vi "CCMWLQuery.vi"(8 "error in (no error)":errorcluster) -> (0 "error out":errorcluster, 1 "Cancel?":bool, 2 "Worklist":string[][](table), 3 "subarray":string[](array[string]))   [LabVIEW 2013, in "main.lvlib" / "ClearCanvasLibrary.lvlib"]
uses:
  ClearCanvasLibrary.lvlib
  <userlib>/_MGI/Error Handling/MGI Suppress Error Code/MGI Suppress Error Code (Scalar).vi
  <vilib>/Utility/cursorutil.llb/Set Cursor (Icon Pict).vi
  <vilib>/Utility/miscctls.llb/LVRowAndColumnTypeDef.ctl
  main.lvlib
  Controls/Enum Save Action Events.ctl
  Controls/SaveDataCluster.ctl
panel:
  in  "TimeEnd":timestamp caption="End" format="%<%x>T"
  in  "TimeStart":timestamp caption="Start" format="%<%x>T"
  in  "SelectPatient":bool
  out "VerificationSCU":bool
  in  "Exit":bool
  in  "queryWorklist":bool
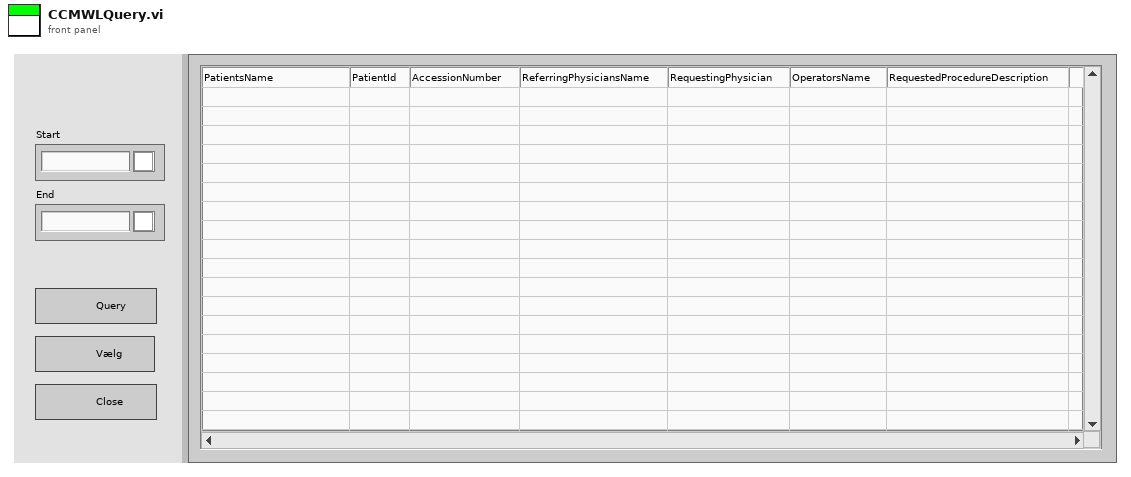
[diagram p1: front panel]
types:
  T1 = typedef "main.lvlib/SaveDataCluster.ctl" = cluster{"HospInfo":cluster{"Name":string, "Address":string, "Department":string}, "Pressure":cluster{"Pressure":dbl}, "DataPath":cluster{"DataPath":path}, "ReportPath":cluster{"Path":path, "Name":string}, "DICOM Info WL":cluster{"port":i32, "AEtitle":string, "host":string, "remoteAE":string}, "DICOM Info PACS":cluster{"port":i32, "AEtitle":string, "host":string, "remoteAE":string}, "ArmCalcMethod":dbl, "itemTags":string[], "DicomEncoding":u16, "JournalType":u16, "General Settings":cluster{"Hyphenation":bool, "Language":u16, "CellStr1":string, "CellStr2":string}, "Dicom Tags":string[][], "BT Serial":cluster{"Serial Number":string, "Side":string, "Ignore?":bool}[], "BT License":cluster{"License":string, "Accepted Serials":string[]}}
  T2 = typedef "main.lvlib/Enum Save Action Events.ctl" = enum16{"LoadReportPath", "SaveReportPath", "Load Graph Path", "Save Graph Path", "LoadDataPath", "SaveDataPath", "Load Template Path", "Save Template Path", "Load PressureFactor", "Save PressureFactor", "Init", "Load Listbox", "Save Listbox", "LoadHospInfo", "SaveHospInfo", "Load DICOM Activation", "Save DICOM Activation", "LoadDICOMInfoWL", "SaveDICOMInfoWL", "LoadDICOMInfoPACS", "SaveDICOMInfoPACS", "Load ArmCalcMethod", "Save ArmCalcMethod", "LoadItemTags", "SaveItemTags", "LoadDICOMEncoding", "SaveDICOMEncoding", "LoadJournalType", "SaveJournalType", "LoadAcqFilterType", "SaveAcqFilterType", "Load Sequence", "Save Sequence", "Load Acquisition Mode", "Save Acquisition Mode", "Load General Settings", "Save General Settings", "Load Language", "Save Language", "Load Dicom Tags", "Save Dicom Tags", "Load BT Serial", "Save BT Serial", "Load BT License", "Save BT License"}
  T3 = typedef "LVRowAndColumnTypeDef.ctl" = cluster{"Row":i32, "Column":i32}
  T4 = cluster{"port":i32, "AEtitle":string, "host":string, "remoteAE":string}
  T5 = cluster{"TimeStart":timestamp, "TimeEnd":timestamp}
  T6 = typedef "LVPoint32TypeDef.ctl" = cluster{"Horizontal":i32, "Vertical":i32}
  T7 = cluster{"port":i32, "AEtitle":string, "remoteAE":string, "host":string}
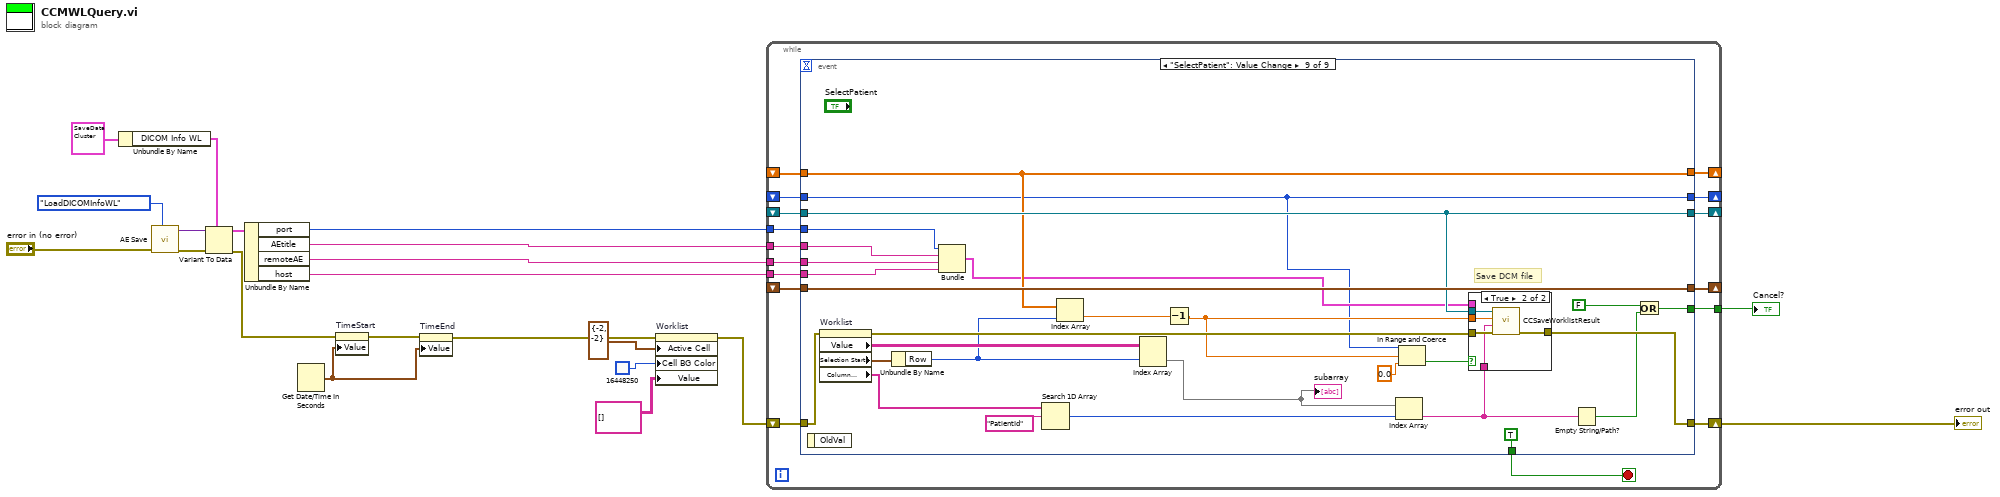
[diagram p0: block diagram]
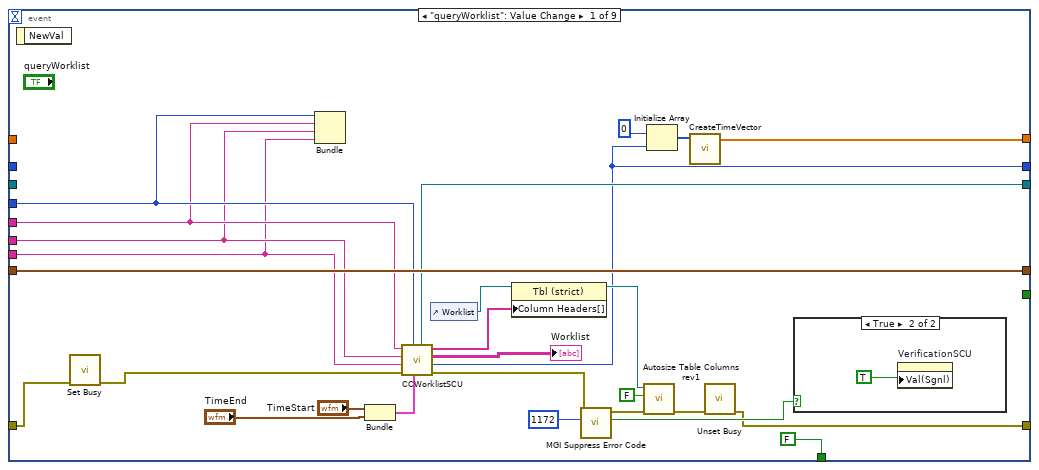
[diagram p2: hidden frame]
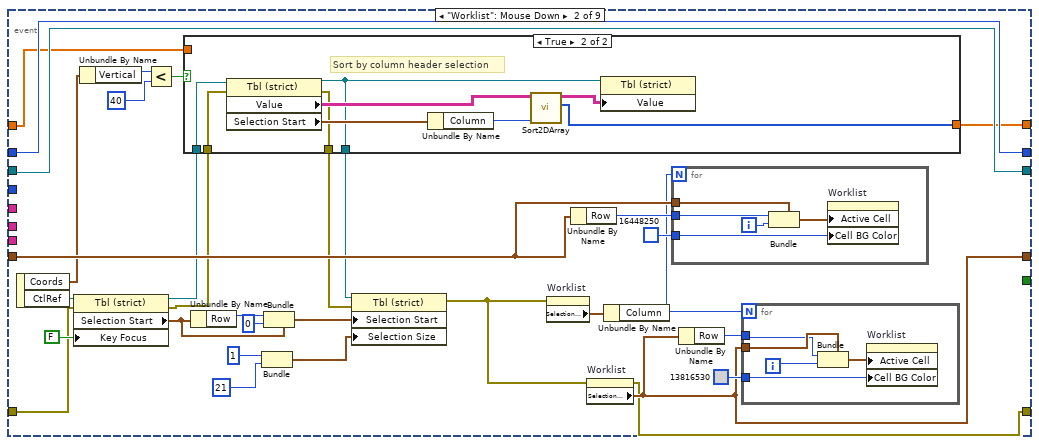
[diagram p4: hidden frame]
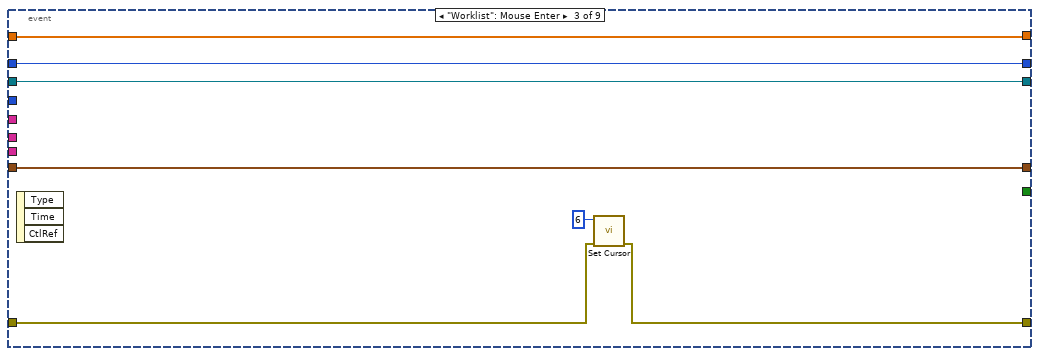
[diagram p6: hidden frame]
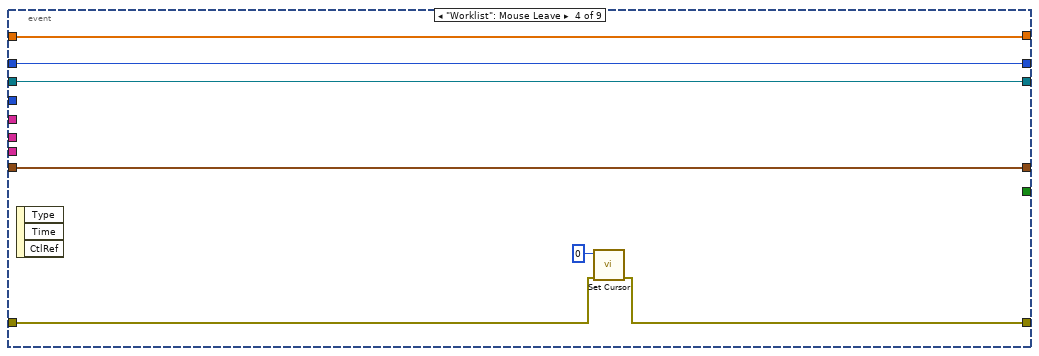
[diagram p7: hidden frame]
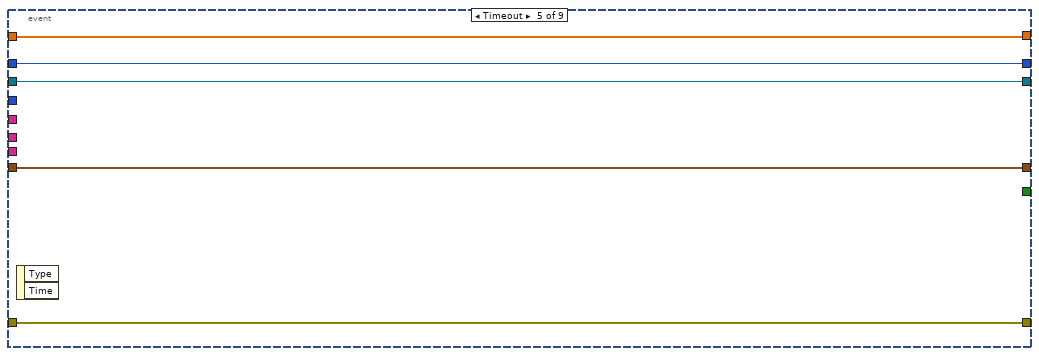
[diagram p8: hidden frame]
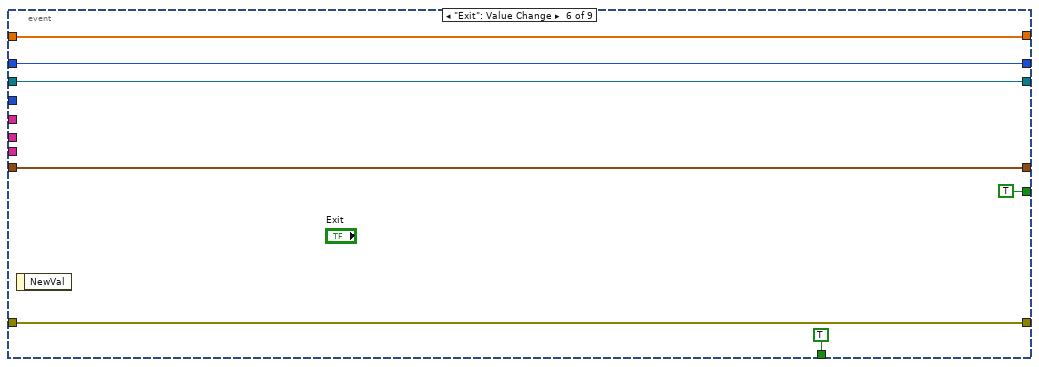
[diagram p9: hidden frame]
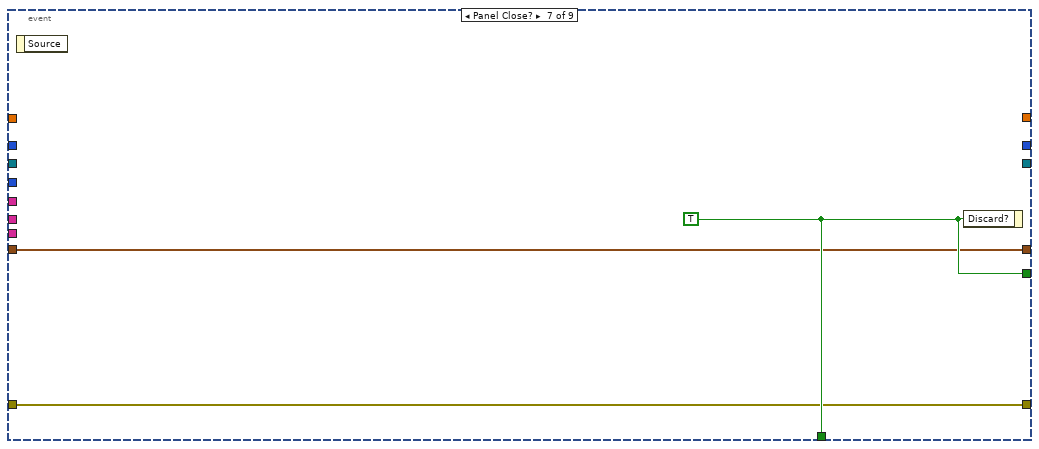
[diagram p10: hidden frame]
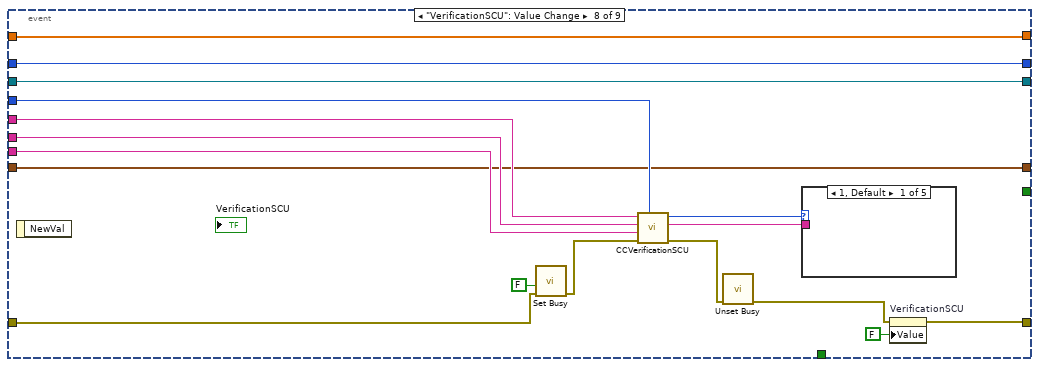
[diagram p11: hidden frame]
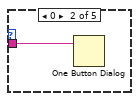
[diagram p12: hidden frame]
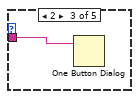
[diagram p13: hidden frame]
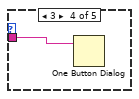
[diagram p14: hidden frame]
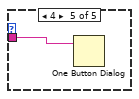
[diagram p15: hidden frame]
diagram:
  n1 = Unbundle By Name(T1 {"HospInfo"={"Name"="", "Address"="", "Department"=""}, "Pressure"={"Pressure"=0.0}, "DataPath"={"DataPath"=path ""}, "ReportPath"={"Path"=path "", "Name"=""}, "DICOM Info WL"={"port"=0, "AEtitle"="", "host"="", "remoteAE"=""}, "DICOM Info PACS"={"port"=0, "AEtitle"="", "host"="", "remoteAE"=""}, "ArmCalcMethod"=0.0, "itemTags"=[], "DicomEncoding"=0, "JournalType"=0, "General Settings"={"Hyphenation"=FALSE, "Language"=0, "CellStr1"="", "CellStr2"=""}, "Dicom Tags"=[], "BT Serial"=[], "BT License"={"License"="", "Accepted Serials"=[]}} ("Data")) -> ("DICOM Info WL"=w11:T4)
  n2 = call "AE Save.vi"("error in (no error)"="error in (no error)", "Action"=Enum_Save_Action_Events."LoadDICOMInfoWL") -> ("error out"=w12:errorcluster, "Anything"=w16:variant)  [unwired: 7 in]
  n3 = Variant To Data(error in=w12, type=w11, Variant=w16) -> (data=w14:T4, error out=w5:errorcluster)
  n4 = Unbundle By Name(w14) -> ("port"=w9:i32, "AEtitle"=w8:string, "remoteAE"=w7:string, "host"=w6:string)
  n5 = Get Date/Time In Seconds() -> (seconds since 1Jan1904=w2:timestamp)
  n6 = property on="TimeStart" class="AbsTime (strict)"(error in=w5, "Value"=w2) -> (error out=w4:errorcluster)  [unwired: 1 in, 1 out]
  n7 = property on="TimeEnd" class="AbsTime (strict)"(error in=w4, "Value"=w2) -> (error out=w3:errorcluster)  [unwired: 1 in, 1 out]
  n8 = property on="Worklist" class="Tbl (strict)"(error in=w3, "Active Cell"=T3 {"Row"=-2, "Column"=-2} ("Active Cell:Active Cell"), "Cell BG Color"=u32 16448250, "Value"=string[][] [] ("Worklist")) -> (error out=w19:errorcluster)  [unwired: 1 in, 1 out]
  n9 = while {
    shift-right: [w36] -> _
    shift-left: _ -> [w35]
    shift-right: [w33] -> w10
    shift-left: w19 -> [w34]
    shift-right: [w32] -> _
    shift-left: _ -> [w31]
    shift-right: [w30] -> _
    shift-left: _ -> [w29]
    tunnel: w9 -> [w28]
    tunnel: w8 -> [w27]
    tunnel: w7 -> [w26]
    tunnel: w6 -> [w25]
    shift-right: [w24] -> _
    shift-left: _ -> [w23]
    tunnel: [w22] -> w1
    stop <- w37 stop-if-true
    n10 = event shown="[8] \"SelectPatient\": Value Change" {
      selector: _ -> [_ _ _ _ _ _ _ _ _]
      dyn-events: _ -> [_ _ _ _ _ _ _ _ _]
      timeout: _ -> [_ _ _ _ _ _ _ _ _]
      tunnel: [FALSE _ _ _ _ TRUE w148 _ TRUE] -> w37
      tunnel: w25 -> [w38 _ _ _ _ _ _ w157 w173]
      tunnel: w26 -> [w39 _ _ _ _ _ _ w158 w172]
      tunnel: w27 -> [w40 _ _ _ _ _ _ w159 w174]
      tunnel: w28 -> [w41 _ _ _ _ _ _ w160 w175]
      tunnel: [w59 w93 w125 w132 w138 w144 w146 w154 w196] -> w36
      tunnel: w35 -> [w59 w92 w125 w132 w138 w144 w146 w154 w196]
      tunnel: w34 -> [w58 w81 w124 w131 w137 w143 w147 w153 w194]
      tunnel: [w57 w80 w123 w130 w137 w143 w147 w152 w191] -> w33
      tunnel: [w56 w79 w122 w129 w136 w142 _ w151 w193] -> w32
      tunnel: w31 -> [_ w79 w122 w129 w136 w142 _ w151 w193]
      tunnel: [w44 w78 w121 w128 w135 w141 _ w150 w170] -> w30
      tunnel: w29 -> [_ w78 w121 w128 w135 w141 _ w150 w170]
      tunnel: [w42 w69 w120 w127 w134 w140 _ w149 w183] -> w24
      tunnel: w23 -> [_ w68 w120 w127 w134 w140 _ w149 w183]
      tunnel: [_ _ _ _ _ TRUE w148 _ w178] -> w22
      event "queryWorklist": Value Change {
        n11 = event-data() -> ()  [unwired: 1 in, 1 out]
        n12 = call <vilib>:"Set Busy.vi"("error in (no error)"=w58) -> ("error out"=w61:errorcluster)  [unwired: 9 in, 1 out]
        n13 = Bundle("port"=w41, "AEtitle"=w40, "remoteAE"=w39, "host"=w38) -> ()  [unwired: 1 in, 1 out]
        n14 = Bundle("TimeStart"="TimeStart", "TimeEnd"="TimeEnd") -> (w55:T5)  [unwired: 1 in]
        n15 = call "CCWorklistSCU.vi"("TimeCluster"=w55, "remotePort"=w41, "error in (no error)"=w61, "remoteHost"=w38, "remoteAE"=w39, "clientAETitle"=w40) -> ("error out"=w60:errorcluster, "patientsRetrieved"=w44:i32, "Worklist"=→"Worklist":string[][], "DicomTags"=w47:string[], "Find"=w56:refnum<k24>)  [unwired: 1 in]
        n16 = control-ref of="Worklist"() -> (w48:refnum<vi>)
        n17 = property class="Tbl (strict)"(reference=w48, "Column Headers[]"=w47) -> (reference out=w46:refnum<vi>)  [unwired: 1 in, 1 out]
        n18 = call-poly <userlib>:"MGI Suppress Error Code.vi"("Error Code"=1172, "Error In"=w60) -> ("Error Supressed?"=w62:bool, "Error Out"=w50:errorcluster)  [unwired: 4 in]
        n19 = call "Autosize Table Columns rev1.vi"("error in (no error)"=w50, "Resize Table?"=FALSE, "Table Ref"=w46) -> ("error out"=w51:errorcluster)  [unwired: 4 in]
        n20 = Initialize Array(0 ("dimension size"), w44) -> (w43:i32[])
        n21 = call "CreateTimeVector.vi"("Array in"=w43) -> ("Array out"=w42:dbl[])  [unwired: 10 in]
        n22 = call <vilib>:"Unset Busy.vi"("error in (no error)"=w51) -> ("error out"=w57:errorcluster)  [unwired: 10 in]
        n23 = case shown="True" w62 {
          frame False {
          }
          frame True {
            n24 = property on="VerificationSCU" class="Bool (strict)"("Val(Sgnl)"=TRUE) -> ()  [unwired: 2 in, 2 out]
          }
        }
      }
      event "Worklist": Mouse Down {
        n25 = event-data() -> ("Coords"=w76:T6, "CtlRef"=w75:refnum<vi>)  [unwired: 1 in]
        n26 = property class="Tbl (strict)"(reference=w75, error in=w81, "Key Focus"=FALSE) -> (reference out=w70:refnum<vi>, error out=w67:errorcluster, "Selection Start"=w90:T3)
        n27 = Unbundle By Name(w76) -> ("Vertical"=w74:i32)
        n28 = Less?(x=w74, y=40) -> (x < y?=w72:bool)
        n29 = case shown="True" w72 {
          tunnel: [w100 w105] -> w71
          tunnel: w70 -> [w100 w104]
          tunnel: [w99 w103] -> w69
          tunnel: w68 -> [w99 _]
          tunnel: w67 -> [w98 w102]
          tunnel: [w98 w101] -> w66
          frame False {
          }
          frame True {
            # "Sort by column header selection"
            n30 = property class="Tbl (strict)"(reference=w104, error in=w102) -> (reference out=w105:refnum<vi>, error out=w101:errorcluster, "Value"=w108:string[][], "Selection Start"=w109:T3)
            n31 = Unbundle By Name(w109) -> ("Column"=w107:i32)
            n32 = call "Sort2DArray.vi"("\"Sort on\" Col/Row indx (0)"=w107, "Array in"=w108) -> ("Sort indices"=w103:i32[], "Sorted Array"=w106:string[][])  [unwired: 7 in, 1 out]
            n33 = property class="Tbl (strict)"(reference=w105, "Value"=w106) -> ()  [unwired: 1 in, 2 out]
          }
        }
        n34 = Unbundle By Name(w90) -> ("Row"=w89:i32)
        n35 = Bundle(1, 21) -> (w85:cluster{i32, i32})  [unwired: 1 in]
        n36 = Bundle(cluster=w90, "Row"=w89, "Column"=0) -> (w86:T3)
        n37 = property class="Tbl (strict)"(reference=w71, error in=w66, "Selection Start"=w86, "Selection Size"=w85) -> (error out=w84:errorcluster)  [unwired: 1 out]
        n38 = property on="Worklist" class="Tbl (strict)"(error in=w84) -> ("Selection Size"=w83:T3)  [unwired: 1 in, 2 out]
        n39 = Unbundle By Name(w92) -> ("Row"=w95:i32)
        n40 = property on="Worklist" class="Tbl (strict)"(error in=w84) -> (error out=w80:errorcluster, "Selection Start"=w93:T3)  [unwired: 1 in, 1 out]
        n41 = Unbundle By Name(w83) -> ("Column"=w82:i32)
        n42 = for {
          N: w82 -> [_]
          tunnel: u32 16448250 -> [w114]
          tunnel: w92 -> [w113]
          tunnel: w95 -> [w112]
          i -> [w111]
          n43 = Bundle(cluster=w113, "Row"=w112, "Column"=w111) -> (w110:T3)
          n44 = property on="Worklist" class="Tbl (strict)"("Active Cell"=w110, "Cell BG Color"=w114) -> ()  [unwired: 2 in, 2 out]
        }
        n45 = Unbundle By Name(w93) -> ("Row"=w96:i32)
        n46 = for {
          N: w82 -> [_]
          tunnel: u32 13816530 -> [w119]
          tunnel: w93 -> [w118]
          tunnel: w96 -> [w117]
          i -> [w116]
          n47 = Bundle(cluster=w118, "Row"=w117, "Column"=w116) -> (w115:T3)
          n48 = property on="Worklist" class="Tbl (strict)"("Active Cell"=w115, "Cell BG Color"=w119) -> ()  [unwired: 2 in, 2 out]
        }
      }
      event "Worklist": Mouse Enter {
        n49 = event-data() -> ()  [unwired: 1 in, 3 out]
        n50 = call-poly <vilib>:"Set Cursor.vi"("error in (no error)"=w124, "icon"=u16 6) -> ("error out"=w123:errorcluster)  [unwired: 8 in, 1 out]
      }
      event "Worklist": Mouse Leave {
        n51 = event-data() -> ()  [unwired: 1 in, 3 out]
        n52 = call-poly <vilib>:"Set Cursor.vi"("error in (no error)"=w131, "icon"=u16 0) -> ("error out"=w130:errorcluster)  [unwired: 8 in, 1 out]
      }
      event Timeout {
        n53 = event-data() -> ()  [unwired: 1 in, 2 out]
      }
      event "Exit": Value Change {
        n54 = event-data() -> ()  [unwired: 1 in, 1 out]
      }
      event Panel Close? {
        w148 = TRUE ("Discard?")
        n55 = event-data() -> ()  [unwired: 1 in, 1 out]
        n56 = event-data("Discard?"=w148) -> ()  [unwired: 1 in, 1 out]
      }
      event "VerificationSCU": Value Change {
        n57 = event-data() -> ()  [unwired: 1 in, 1 out]
        n58 = call <vilib>:"Set Busy.vi"("error in (no error)"=w153, "disable click? (T)"=FALSE) -> ("error out"=w163:errorcluster)  [unwired: 8 in, 1 out]
        n59 = call "CCVerificationSCU.vi"("remotePort"=w160, "error in (no error)"=w163, "remoteHost"=w157, "remoteAE"=w158, "clientAETitle"=w159) -> ("error out"=w162:errorcluster, "FailureDescription"=w164:string, "Result"=w165:i32)  [unwired: 4 in]
        n60 = call <vilib>:"Unset Busy.vi"("error in (no error)"=w162) -> ("error out"=w156:errorcluster)  [unwired: 10 in]
        n61 = case shown="1, Default" w165 {
          tunnel: w164 -> [_ w166 w167 w168 w169]
          frame 1, Default {
          }
          frame 0 {
            n62 = One Button Dialog(message=w166) -> ()  [unwired: 1 in, 1 out]
          }
          frame 2 {
            n63 = One Button Dialog(message=w167) -> ()  [unwired: 1 in, 1 out]
          }
          frame 3 {
            n64 = One Button Dialog(message=w168) -> ()  [unwired: 1 in, 1 out]
          }
          frame 4 {
            n65 = One Button Dialog(message=w169) -> ()  [unwired: 1 in, 1 out]
          }
        }
        n66 = property on="VerificationSCU" class="Bool (strict)"(error in=w156, "Value"=FALSE ("Boolean")) -> (error out=w152:errorcluster)  [unwired: 1 in, 1 out]
      }
      event "SelectPatient": Value Change {
        # "Save DCM file"
        n67 = event-data() -> ()  [unwired: 1 in, 1 out]
        n68 = property on="Worklist" class="Tbl (strict)"(error in=w194) -> (error out=w192:errorcluster, "Value"=w188:string[][], "Selection Start"=w197:T3, "Column Headers[]"=w184:string[])  [unwired: 1 in, 1 out]
        n69 = Unbundle By Name(w197) -> ("Row"=w182:i32)
        n70 = Bundle("port"=w175, "AEtitle"=w174, "remoteAE"=w172, "host"=w173) -> (w171:T7)  [unwired: 1 in]
        n71 = Search 1D Array(1D array=w184, element="PatientId") -> (index of element=w186:i32)  [unwired: 1 in]
        n72 = Index Array(array=w183, index=w182) -> (element=w180:dbl)
        n73 = Index Array(array=w188, index (row)=w182) -> (element=w185:string[])  [unwired: 1 in]
        "subarray" <- w185
        n74 = Decrement(x=w180) -> (x-1=w181:dbl)
        n75 = Index Array(array=w185, index=w186) -> (element=w179:string)
        n76 = In Range and Coerce(upper limit=w170, x=w181, lower limit=0.0) -> (In Range?=w189:bool)  [unwired: 1 out]
        n77 = case shown="True" w189 {
          tunnel: w193 -> [_ w203]
          tunnel: w192 -> [w198 w201]
          tunnel: [w198 w202] -> w191
          tunnel: w181 -> [_ w200]
          tunnel: w179 -> [_ w199]
          tunnel: w171 -> [_ _]
          frame False {
          }
          frame True {
            n78 = call "CCSaveWorklistResult.vi"("error in (no error)"=w201, "patientID"=w199, "index"=w200, "Find"=w203) -> ("error out"=w202:errorcluster)  [unwired: 7 in]
          }
        }
        n79 = Empty String/Path?(string/path=w179) -> (empty?=w176:bool)
        n80 = Or(x=FALSE, y=w176) -> (x .or. y?=w178:bool)
      }
    }
  }
  "error out" <- w10
  "Cancel?" <- w1
